vi "Process PA GPS Data.vi"(11 "RDS State in":refnum<class "RDS State.lvclass">) -> (3 "RDS State out":refnum<class "RDS State.lvclass">)   [LabVIEW 2015, in "RDS Child Messages.lvlib" / "RDS State.lvclass"]
uses:
  RDS State.lvclass
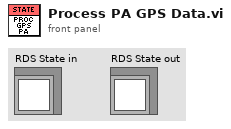
[diagram p1: front panel]
types:
  T1 = typedef "NMEA.lvlib/NMEA_GPRMC-data.ctl" = cluster{"TimeStamp":timestamp, "Validity":bool, "Latitude":dbl, "Latitude-Direction":T2, "Longitude":dbl, "Longitude-Direction":T3, "Speed in knots":dbl, "True course":dbl, "Date Stamp":timestamp, "Magnetic Variation (East/West)":dbl, "GPS Latitude":ext, "GPS Longitude":ext}
  T2 = typedef "NMEA.lvlib/NMEA_LatitudeDirection.ctl" = enum16{"", "North", "South"}
  T3 = typedef "NMEA.lvlib/NMEA_LongitudeDirection.ctl" = enum16{"", "East", "West"}
  T4 = typedef "Processed PA Block.ctl" = cluster{"GPS Heading":dbl, "GPS Speed":dbl, "GPS Latitude":ext, "GPS Longitude":ext, "Compass heading":dbl, "Pitch":dbl, "Roll":dbl}
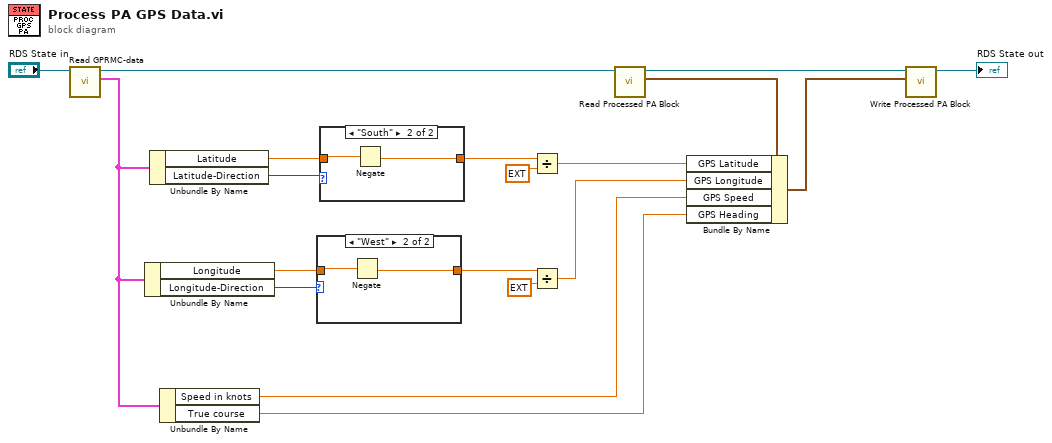
[diagram p0: block diagram]
diagram:
  n1 = call "Read GPRMC-data.vi"("RDS State in"="RDS State in") -> ("GPRMC-data"=w5:T1, "RDS State out"=w16:refnum<class "RDS State.lvclass">)  [unwired: 8 in, 1 out]
  n2 = Unbundle By Name(w5) -> ("Longitude"=w11:dbl, "Longitude-Direction"=w10:T3)
  n3 = Unbundle By Name(w5) -> ("Latitude"=w14:dbl, "Latitude-Direction"=w15:T2)
  n4 = Unbundle By Name(w5) -> ("Speed in knots"=w4:dbl, "True course"=w3:dbl)
  n5 = case shown="\"West\"" w10 {
    tunnel: w11 -> [w20 w22]
    tunnel: [w20 w21] -> w8
    frame "East", Default {
    }
    frame "West" {
      n6 = Negate(x=w22) -> (-x=w21:dbl)
    }
  }
  n7 = case shown="\"South\"" w15 {
    tunnel: w14 -> [w23 w25]
    tunnel: [w23 w24] -> w12
    frame "North", Default {
    }
    frame "South" {
      n8 = Negate(x=w25) -> (-x=w24:dbl)
    }
  }
  n9 = Divide(x=w12, y=ext 100.0) -> (x/y=w1:ext)
  n10 = Divide(x=w8, y=ext 100.0) -> (x/y=w2:ext)
  n11 = call "Read Processed PA Block.vi"("RDS State in"=w16) -> ("Processed PA Block"=w7:T4, "RDS State out"=w18:refnum<class "RDS State.lvclass">)  [unwired: 8 in, 1 out]
  n12 = Bundle By Name(cluster=w7, "GPS Latitude"=w1, "GPS Longitude"=w2, "GPS Speed"=w4, "GPS Heading"=w3) -> (w6:T4)
  n13 = call "Write Processed PA Block.vi"("Processed PA Block"=w6, "RDS State in"=w18) -> ("RDS State out"=→"RDS State out":refnum<class "RDS State.lvclass">)  [unwired: 8 in, 1 out]
